vi "PTSequencer.ProcCases.vi"(0 "i ref in":refnum<vi>, 1 "selector":string, 2 "Data":T3, 3 "call cluster":T1={"Object"="", "Selector"="", "CallType"=enum."synchronous", "Async Object"="", "Async Selector"="", "Data Descriptor"="", "Data"=[], "Error #"=0, "Expire"=0}, 5 "error in (no error)":errorcluster) -> (14 "i ref out":refnum<vi>, 17 "answer cluster":T1={"Object"="", "Selector"="", "CallType"=enum."synchronous", "Async Object"="", "Async Selector"="", "Data Descriptor"="", "Data"=[], "Error #"=0, "Expire"=0}, 19 "error out":errorcluster)   [LabVIEW 2014, in "PTSequencer.lvlib"]
uses:
  PTSequencer.lvlib
  CSCore/CSSystem/CoreDefs/CoreDefs.rawDataType.ctl
  CSCore/CSSystem/CoreDefs/CoreDefs.call_type.ctl
  CSCore/BaseProcess/BaseProcess.descriptor string definition.ctl
  CSCore/CSSystem/CoreLib/CoreLib.string 2 byte array.vi
  CSCore/CSSystem/CoreLib/CoreLib.byte array 2 string.vi
  CSCore/BaseProcess/BaseProcess.lvlib
  CSCore/CAEObj/CAEObj.lvlib
  CSCore/CSSystem/CoreLib/CoreLib.lvlib
  CSCore/BaseSM/BaseSM.lvlib
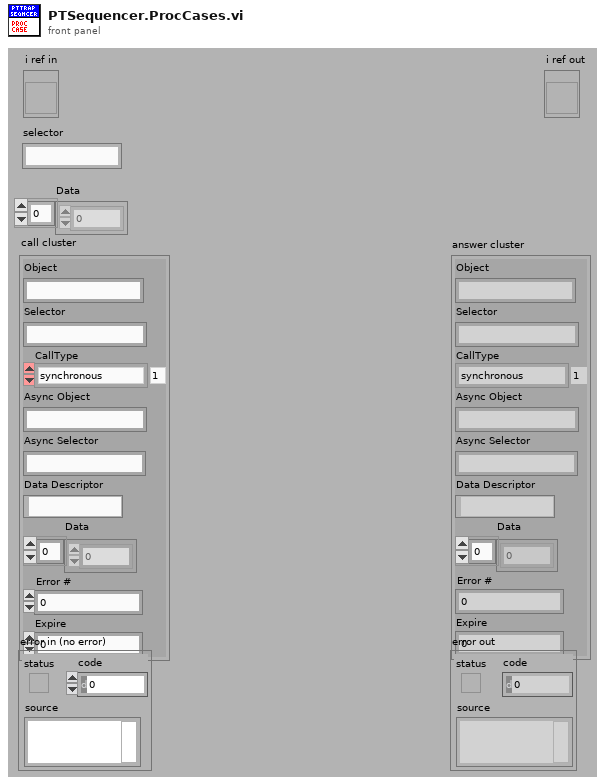
[diagram p1: front panel]
types:
  T1 = typedef "CoreDefs.call_type.ctl" = cluster{"Object":string, "Selector":string, "CallType":enum16{"simple", "synchronous", "asynchronous"}, "Async Object":string, "Async Selector":string, "Data Descriptor":T2, "Data":T3, "Error #":i32, "Expire":u32}
  T2 = typedef "BaseProcess.lvlib/BaseProcess.descriptor string definition.ctl" = string
  T3 = typedef "CoreDefs.rawDataType.ctl" = i8[]
  T4 = typedef "PTSequencer.lvlib/PTSequencer.i attribute.ctl" = cluster{"subsequence":bool, "mode":T5, "i step":i32, "nofLoops":i32, "i loop":i32, "Running":bool, "Paused":bool, "step done":bool, "loop done":bool, "seq done":bool, "DIM IDs":cluster{"step done":i32, "loop done":i32, "seq done":i32, "i step":i32, "i loop":i32}, "use stop conditions":bool, "stop conditions":T6[], "Step List":T7[], "DIM subsriptions":string[], "stop cond indexes":i32[], "step cond indexes":cluster{"step condition IDs":cluster{"step ID":i32, "condition ID":i32}[]}[], "Delay Start Time":timestamp, "status":string, "stopping":bool}
  T5 = typedef "PTSequencer.lvlib/PTSequencer.mode.ctl" = enum16{"single", "loop", "for loop"}
  T6 = typedef "PTSequencer.lvlib/PTSequencer.DIM service condition.ctl" = cluster{"DIM service":string, "descr":string, "nomValue":T3, "actValue":T3, "matched":bool, "DIM Status":cluster{"no link":bool, "quality":i32, "Time Stamp":timestamp}}
  T7 = typedef "PTSequencer.lvlib/PTSequencer.step.ctl" = cluster{"description":string, "object parameters":cluster{"object":string, "selector":string, "descriptor":string, "data":T3, "subsequence":bool, "call mode":enum16{"Simple DIM", "Synchronous"}, "data in":T3}, "result action":cluster{"check":bool, "passed":enum16{"Next", "Previous", "Repeat", "Jump"}, "failed":enum16{"Next", "Previous", "Repeat", "Jump"}, "jumpID_passed":i32, "jumpID_failed":i32}, "conditions":T6[], "fulfilled ":bool, "use delay":bool, "delay time (s)":dbl, "ID":i32}
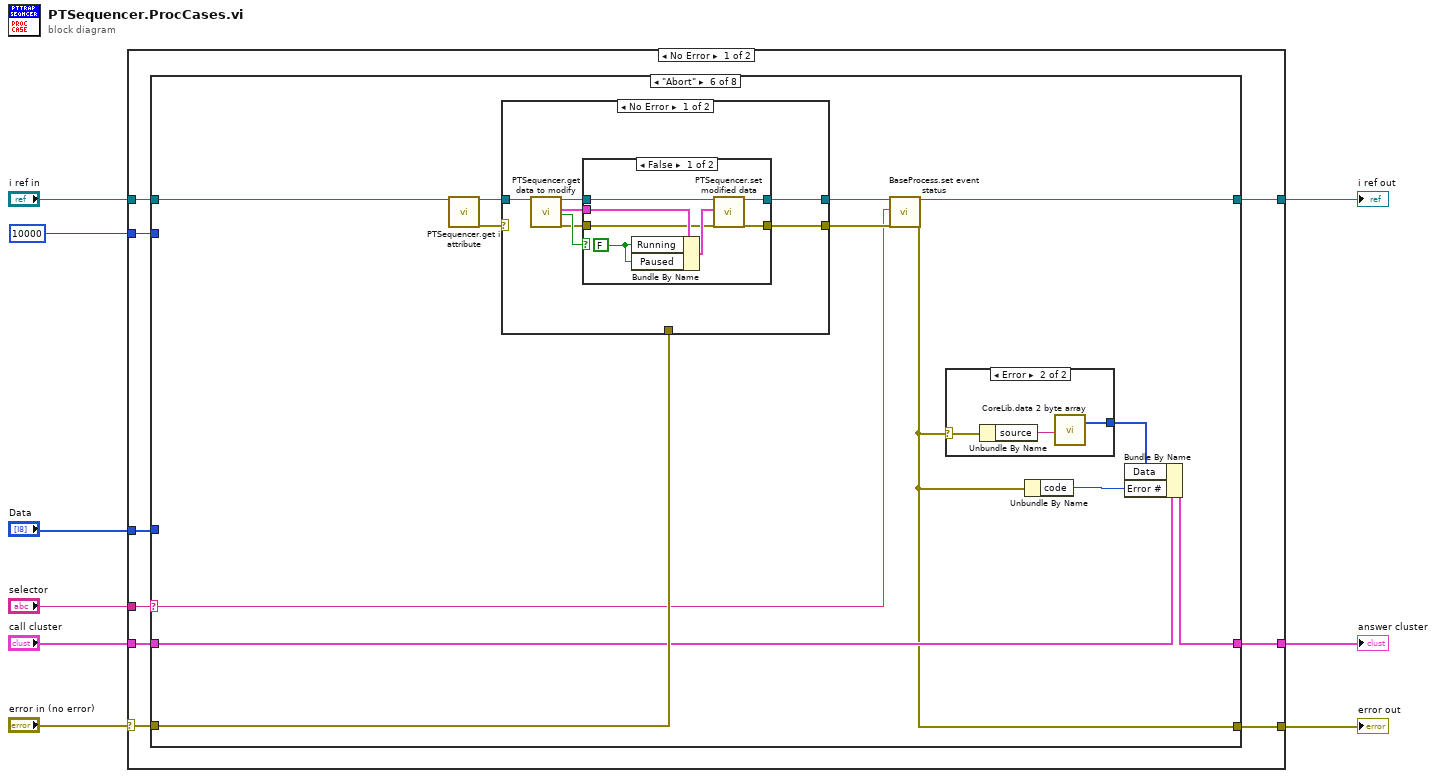
[diagram p0: block diagram]
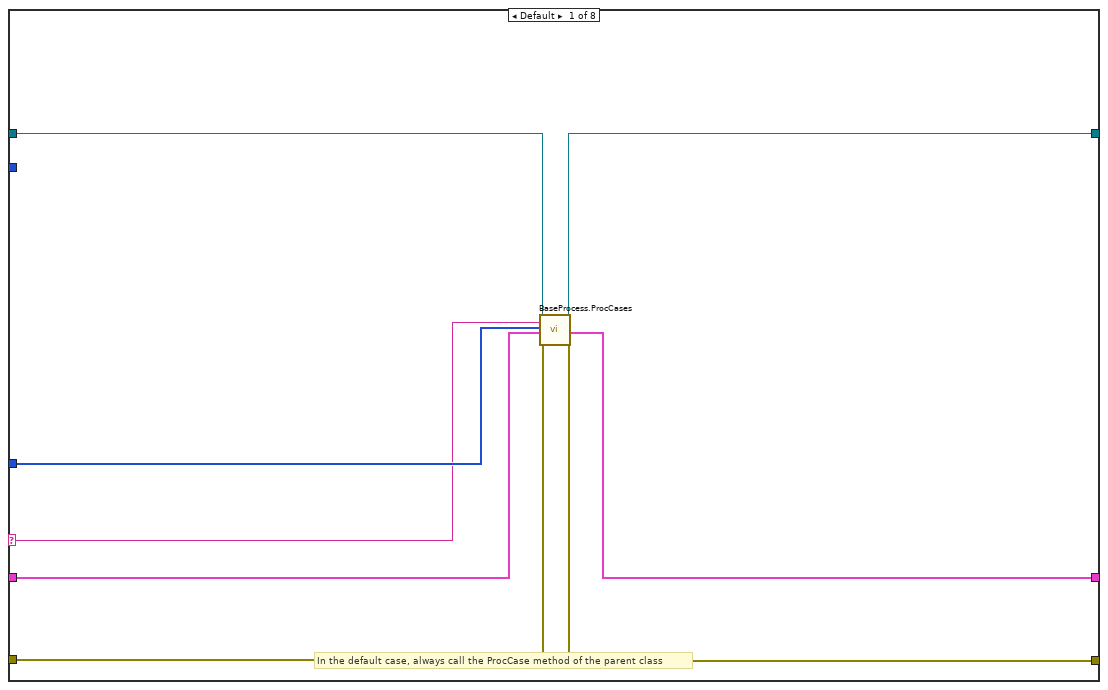
[diagram p2: hidden frame]
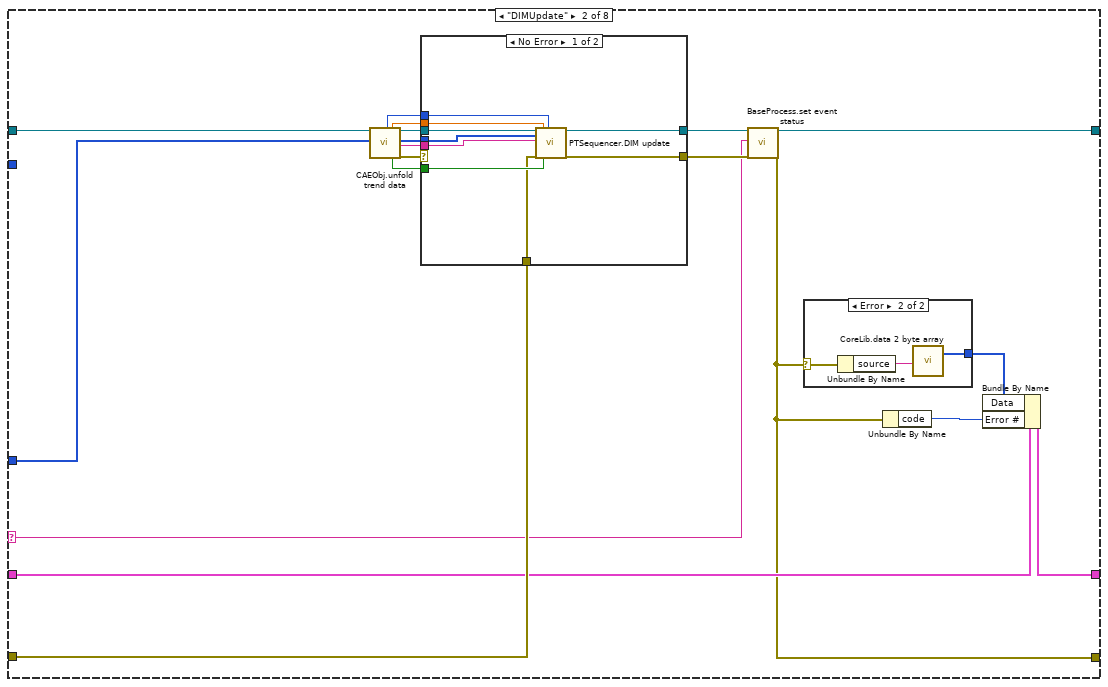
[diagram p3: hidden frame]
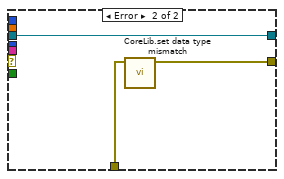
[diagram p5: hidden frame]
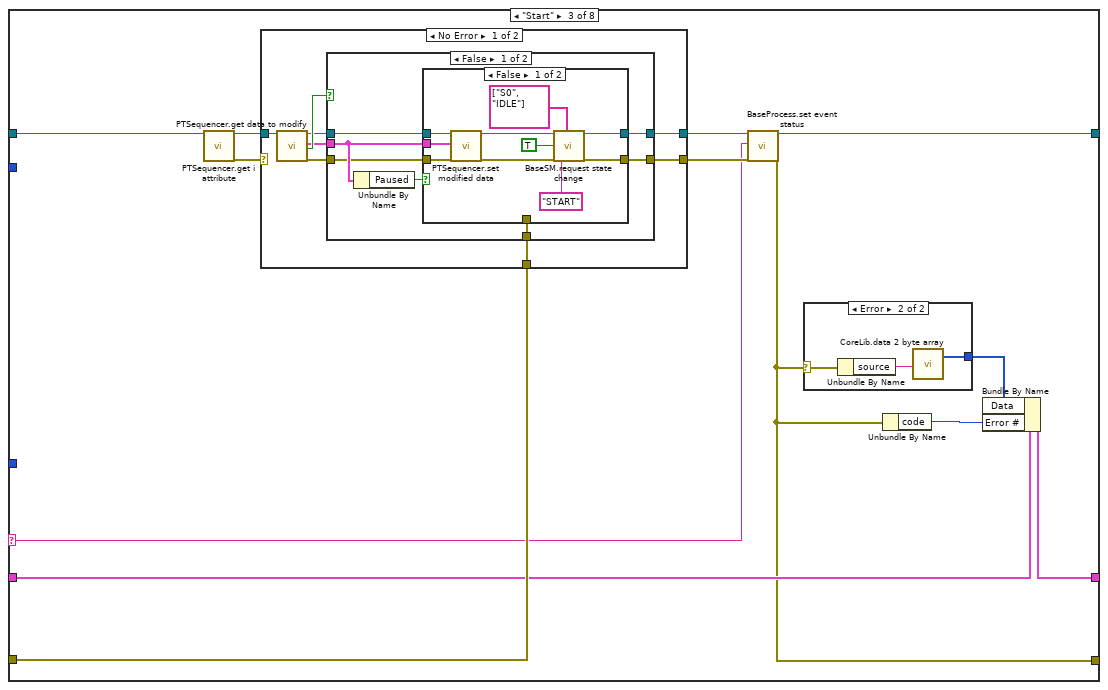
[diagram p6: hidden frame]
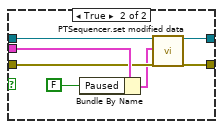
[diagram p8: hidden frame]
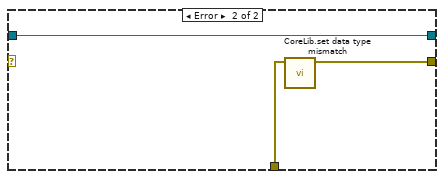
[diagram p10: hidden frame]
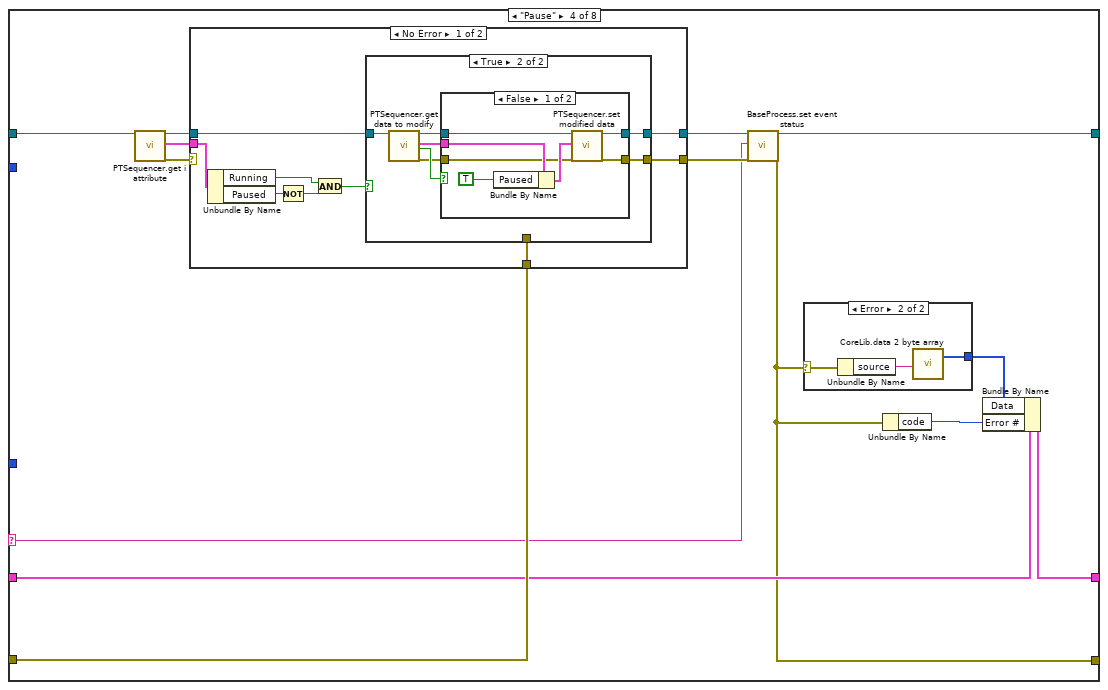
[diagram p11: hidden frame]
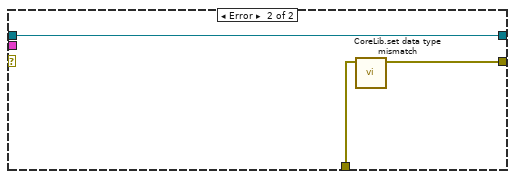
[diagram p15: hidden frame]
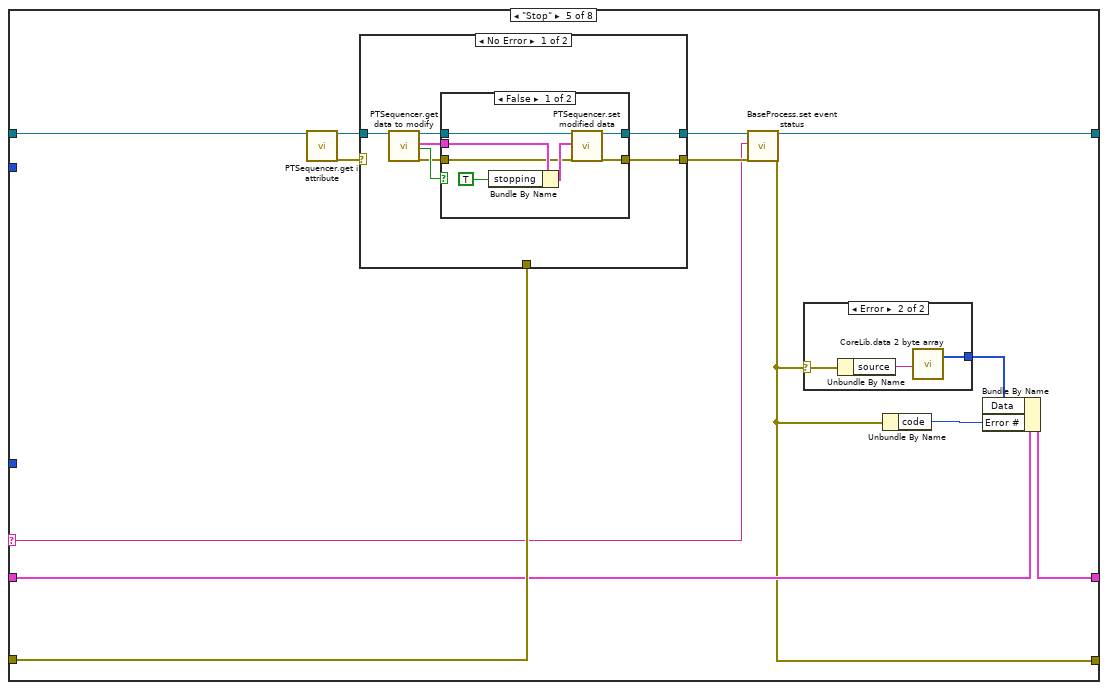
[diagram p16: hidden frame]
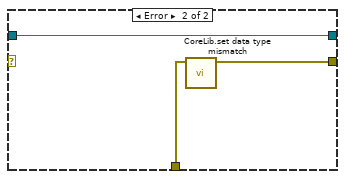
[diagram p19: hidden frame]
diagram:
  n1 = case shown="No Error" "error in (no error)" {
    selector: "error in (no error)" -> [w10 w281]
    tunnel: "selector" -> [w18 _]
    tunnel: [w17 w282] -> w8
    tunnel: "Data" -> [w16 _]
    tunnel: "call cluster" -> [w15 w282]
    tunnel: "i ref in" -> [w14 w283]
    tunnel: [w13 w283] -> w4
    tunnel: [w12 w281] -> w3
    tunnel: 10000 -> [w11 _]
    frame No Error {
      n2 = case shown="\"Abort\"" w18 {
        selector: w18 -> [w20 w30 w65 w119 w165 w200 w240 w265]
        tunnel: w16 -> [w21 w39 _ _ _ _ _ _]
        tunnel: w14 -> [w19 w29 w62 w116 w162 w197 w238 w263]
        tunnel: [w26 w28 w64 w118 w164 w199 w239 w264] -> w13
        tunnel: w15 -> [w22 w33 w68 w122 w168 w203 w234 w259]
        tunnel: [w23 w32 w67 w121 w167 w202 w242 w267] -> w17
        tunnel: w10 -> [w25 w36 w71 w125 w171 w206 w235 w260]
        tunnel: [w24 w31 w66 w120 w166 w201 w241 w266] -> w12
        tunnel: w11 -> [_ _ _ _ _ _ _ _]
        frame Default {
          # "In the default case, always call the ProcCase method of the parent class"
          n3 = call "BaseProcess.ProcCases.vi"("i ref in"=w19, "selector"=w20, "Data"=w21, "call cluster"=w22, "error in (no error)"=w25) -> ("i ref out"=w26:refnum<vi>, "answer cluster"=w23:T1, "error out"=w24:errorcluster)  [unwired: 12 in]
        }
        frame "DIMUpdate" {
          n4 = call "CAEObj.unfold trend data.vi"("i ref in"=w29, "raw trend data"=w39) -> ("quality"=w42:i32, "timeStamp"=w43:dbl, "no link"=w41:bool, "i ref out"=w27:refnum<vi>, "data"=w44:i8[], "serviceName"=w40:string, "error out"=w45:errorcluster)  [unwired: 9 in, 2 out]
          n5 = case shown="No Error" w45 {
            tunnel: w44 -> [w52 _]
            tunnel: w43 -> [w50 _]
            tunnel: w42 -> [w51 _]
            tunnel: [w55 w60] -> w34
            tunnel: w27 -> [w57 w59]
            tunnel: [w56 w59] -> w35
            tunnel: w41 -> [w54 _]
            tunnel: w40 -> [w53 _]
            tunnel: w36 -> [w49 w58]
            frame No Error {
              n6 = call "PTSequencer.DIM update.vi"("i ref in"=w57, "data"=w52, "serviceName"=w53, "error in (no error)"=w49, "Time Stamp"=w50, "no link"=w54, "quality"=w51) -> ("i ref out"=w56:refnum<vi>, "error out"=w55:errorcluster)  [unwired: 11 in]
            }
            frame Error {
              n7 = call "CoreLib.set data type mismatch.vi"("error in (no error)"=w58) -> ("error out"=w60:errorcluster)  [unwired: 18 in]
            }
          }
          n8 = call "BaseProcess.set event status.vi"("i ref in"=w35, "EventStatus"=w30, "error in (no error)"=w34) -> ("i ref out"=w28:refnum<vi>, "error out"=w31:errorcluster)  [unwired: 14 in, 1 out]
          n9 = case shown="Error" w31 {
            selector: w31 -> [_ w48]
            tunnel: [_ w46] -> w37
            frame No Error {
            }
            frame Error {
              n10 = Unbundle By Name(w48) -> ("source"=w47:string)
              n11 = call-poly "CoreLib.data 2 byte array.vi"("string"=w47) -> ("byteArray out"=w46:T3)  [unwired: 18 in]
            }
          }
          n12 = Unbundle By Name(w31) -> ("code"=w38:i32)
          n13 = Bundle By Name(cluster=w33, "Data"=w37, "Error #"=w38) -> (w32:T1)
        }
        frame "Start" {
          n14 = call "PTSequencer.get i attribute.vi"("i ref in"=w62) -> ("i ref out"=w61:refnum<vi>, "error out"=w63:errorcluster)  [unwired: 16 in, 1 out]
          n15 = case shown="No Error" w63 {
            tunnel: [w83 w113] -> w69
            tunnel: w61 -> [w81 w112]
            tunnel: [w84 w112] -> w70
            tunnel: w71 -> [w82 w111]
            frame No Error {
              n16 = call "PTSequencer.get data to modify.vi"("i ref in"=w81) -> ("i ref out"=w79:refnum<vi>, "i attribute"=w77:T4, "timed out"=w80:bool, "error out"=w78:errorcluster)  [unwired: 15 in]
              n17 = case shown="False" w80 {
                tunnel: [w91 w110] -> w84
                tunnel: [w90 w109] -> w83
                tunnel: w82 -> [w89 _]
                tunnel: w79 -> [w87 w110]
                tunnel: w78 -> [w85 w109]
                tunnel: w77 -> [w86 _]
                frame False {
                  n18 = Unbundle By Name(w86) -> ("Paused"=w88:bool)
                  n19 = case shown="False" w88 {
                    tunnel: [w98 w108] -> w91
                    tunnel: [w97 w104] -> w90
                    tunnel: w89 -> [_ _]
                    tunnel: w87 -> [w96 w107]
                    tunnel: w86 -> [w95 w106]
                    tunnel: w85 -> [w94 w105]
                    frame False {
                      n20 = call "PTSequencer.set modified data.vi"("i ref in"=w96, "CLASS.i attribute"=w95, "error in (no error)"=w94) -> ("i ref out"=w92:refnum<vi>, "error out"=w93:errorcluster)  [unwired: 15 in]
                      n21 = call "BaseSM.request state change.vi"("i ref in"=w92, "change"=TRUE, "error in (no error)"=w93, "requested state"="START", "allowed current states"=string[] ["S0", "IDLE"]) -> ("i ref out"=w98:refnum<vi>, "error out"=w97:errorcluster)  [unwired: 11 in, 2 out]
                    }
                    frame True {
                      n22 = Bundle By Name(cluster=w106, "Paused"=FALSE) -> (w103:T4)
                      n23 = call "PTSequencer.set modified data.vi"("i ref in"=w107, "CLASS.i attribute"=w103, "error in (no error)"=w105) -> ("i ref out"=w108:refnum<vi>, "error out"=w104:errorcluster)  [unwired: 15 in]
                    }
                  }
                }
                frame True {
                }
              }
            }
            frame Error {
              n24 = call "CoreLib.set data type mismatch.vi"("error in (no error)"=w111) -> ("error out"=w113:errorcluster)  [unwired: 18 in]
            }
          }
          n25 = call "BaseProcess.set event status.vi"("i ref in"=w70, "EventStatus"=w65, "error in (no error)"=w69) -> ("i ref out"=w64:refnum<vi>, "error out"=w66:errorcluster)  [unwired: 14 in, 1 out]
          n26 = case shown="Error" w66 {
            selector: w66 -> [_ w76]
            tunnel: [_ w74] -> w72
            frame No Error {
            }
            frame Error {
              n27 = Unbundle By Name(w76) -> ("source"=w75:string)
              n28 = call-poly "CoreLib.data 2 byte array.vi"("string"=w75) -> ("byteArray out"=w74:T3)  [unwired: 18 in]
            }
          }
          n29 = Unbundle By Name(w66) -> ("code"=w73:i32)
          n30 = Bundle By Name(cluster=w68, "Data"=w72, "Error #"=w73) -> (w67:T1)
        }
        frame "Pause" {
          n31 = call "PTSequencer.get i attribute.vi"("i ref in"=w116) -> ("i ref out"=w115:refnum<vi>, "i attribute"=w114:T4, "error out"=w117:errorcluster)  [unwired: 16 in]
          n32 = case shown="No Error" w117 {
            tunnel: [w138 w160] -> w123
            tunnel: w115 -> [w131 w159]
            tunnel: [w139 w159] -> w124
            tunnel: w125 -> [w137 w158]
            tunnel: w114 -> [w136 _]
            frame No Error {
              n33 = Unbundle By Name(w136) -> ("Running"=w133:bool, "Paused"=w135:bool)
              n34 = Not(x=w135) -> (.not. x?=w134:bool)
              n35 = And(x=w133, y=w134) -> (x .and. y?=w132:bool)
              n36 = case shown="True" w132 {
                tunnel: w131 -> [w141 w148]
                tunnel: [w141 w145] -> w139
                tunnel: [w140 w142] -> w138
                tunnel: w137 -> [w140 _]
                frame False {
                }
                frame True {
                  n37 = call "PTSequencer.get data to modify.vi"("i ref in"=w148) -> ("i ref out"=w146:refnum<vi>, "i attribute"=w147:T4, "timed out"=w144:bool, "error out"=w143:errorcluster)  [unwired: 15 in]
                  n38 = case shown="False" w144 {
                    tunnel: w147 -> [w155 _]
                    tunnel: w146 -> [w154 w157]
                    tunnel: [w153 w157] -> w145
                    tunnel: w143 -> [w150 w156]
                    tunnel: [w149 w156] -> w142
                    frame False {
                      n39 = Bundle By Name(cluster=w155, "Paused"=TRUE) -> (w151:T4)
                      n40 = call "PTSequencer.set modified data.vi"("i ref in"=w154, "CLASS.i attribute"=w151, "error in (no error)"=w150) -> ("i ref out"=w153:refnum<vi>, "error out"=w149:errorcluster)  [unwired: 15 in]
                    }
                    frame True {
                    }
                  }
                }
              }
            }
            frame Error {
              n41 = call "CoreLib.set data type mismatch.vi"("error in (no error)"=w158) -> ("error out"=w160:errorcluster)  [unwired: 18 in]
            }
          }
          n42 = call "BaseProcess.set event status.vi"("i ref in"=w124, "EventStatus"=w119, "error in (no error)"=w123) -> ("i ref out"=w118:refnum<vi>, "error out"=w120:errorcluster)  [unwired: 14 in, 1 out]
          n43 = case shown="Error" w120 {
            selector: w120 -> [_ w130]
            tunnel: [_ w128] -> w126
            frame No Error {
            }
            frame Error {
              n44 = Unbundle By Name(w130) -> ("source"=w129:string)
              n45 = call-poly "CoreLib.data 2 byte array.vi"("string"=w129) -> ("byteArray out"=w128:T3)  [unwired: 18 in]
            }
          }
          n46 = Unbundle By Name(w120) -> ("code"=w127:i32)
          n47 = Bundle By Name(cluster=w122, "Data"=w126, "Error #"=w127) -> (w121:T1)
        }
        frame "Stop" {
          n48 = call "PTSequencer.get i attribute.vi"("i ref in"=w162) -> ("i ref out"=w161:refnum<vi>, "error out"=w163:errorcluster)  [unwired: 16 in, 1 out]
          n49 = case shown="No Error" w163 {
            tunnel: [w177 w195] -> w169
            tunnel: w161 -> [w183 w194]
            tunnel: [w182 w194] -> w170
            tunnel: w171 -> [_ w193]
            frame No Error {
              n50 = call "PTSequencer.get data to modify.vi"("i ref in"=w183) -> ("i ref out"=w180:refnum<vi>, "i attribute"=w181:T4, "timed out"=w179:bool, "error out"=w178:errorcluster)  [unwired: 15 in]
              n51 = case shown="False" w179 {
                tunnel: w181 -> [w190 _]
                tunnel: w180 -> [w189 w192]
                tunnel: [w188 w192] -> w182
                tunnel: w178 -> [w185 w191]
                tunnel: [w184 w191] -> w177
                frame False {
                  n52 = Bundle By Name(cluster=w190, "stopping"=TRUE ("Paused")) -> (w186:T4)
                  n53 = call "PTSequencer.set modified data.vi"("i ref in"=w189, "CLASS.i attribute"=w186, "error in (no error)"=w185) -> ("i ref out"=w188:refnum<vi>, "error out"=w184:errorcluster)  [unwired: 15 in]
                }
                frame True {
                }
              }
            }
            frame Error {
              n54 = call "CoreLib.set data type mismatch.vi"("error in (no error)"=w193) -> ("error out"=w195:errorcluster)  [unwired: 18 in]
            }
          }
          n55 = call "BaseProcess.set event status.vi"("i ref in"=w170, "EventStatus"=w165, "error in (no error)"=w169) -> ("i ref out"=w164:refnum<vi>, "error out"=w166:errorcluster)  [unwired: 14 in, 1 out]
          n56 = case shown="Error" w166 {
            selector: w166 -> [_ w176]
            tunnel: [_ w174] -> w172
            frame No Error {
            }
            frame Error {
              n57 = Unbundle By Name(w176) -> ("source"=w175:string)
              n58 = call-poly "CoreLib.data 2 byte array.vi"("string"=w175) -> ("byteArray out"=w174:T3)  [unwired: 18 in]
            }
          }
          n59 = Unbundle By Name(w166) -> ("code"=w173:i32)
          n60 = Bundle By Name(cluster=w168, "Data"=w172, "Error #"=w173) -> (w167:T1)
        }
        frame "Abort" {
          n61 = call "PTSequencer.get i attribute.vi"("i ref in"=w197) -> ("i ref out"=w196:refnum<vi>, "error out"=w198:errorcluster)  [unwired: 16 in, 1 out]
          n62 = case shown="No Error" w198 {
            tunnel: [w212 w230] -> w204
            tunnel: w196 -> [w218 w229]
            tunnel: [w217 w229] -> w205
            tunnel: w206 -> [_ w228]
            frame No Error {
              n63 = call "PTSequencer.get data to modify.vi"("i ref in"=w218) -> ("i ref out"=w215:refnum<vi>, "i attribute"=w216:T4, "timed out"=w214:bool, "error out"=w213:errorcluster)  [unwired: 15 in]
              n64 = case shown="False" w214 {
                tunnel: w216 -> [w225 _]
                tunnel: w215 -> [w224 w227]
                tunnel: [w223 w227] -> w217
                tunnel: w213 -> [w221 w226]
                tunnel: [w220 w226] -> w212
                frame False {
                  w219 = FALSE ("Paused")
                  n65 = Bundle By Name(cluster=w225, "Running"=w219, "Paused"=w219) -> (w222:T4)
                  n66 = call "PTSequencer.set modified data.vi"("i ref in"=w224, "CLASS.i attribute"=w222, "error in (no error)"=w221) -> ("i ref out"=w223:refnum<vi>, "error out"=w220:errorcluster)  [unwired: 15 in]
                }
                frame True {
                }
              }
            }
            frame Error {
              n67 = call "CoreLib.set data type mismatch.vi"("error in (no error)"=w228) -> ("error out"=w230:errorcluster)  [unwired: 18 in]
            }
          }
          n68 = call "BaseProcess.set event status.vi"("i ref in"=w205, "EventStatus"=w200, "error in (no error)"=w204) -> ("i ref out"=w199:refnum<vi>, "error out"=w201:errorcluster)  [unwired: 14 in, 1 out]
          n69 = case shown="Error" w201 {
            selector: w201 -> [_ w211]
            tunnel: [_ w209] -> w207
            frame No Error {
            }
            frame Error {
              n70 = Unbundle By Name(w211) -> ("source"=w210:string)
              n71 = call-poly "CoreLib.data 2 byte array.vi"("string"=w210) -> ("byteArray out"=w209:T3)  [unwired: 18 in]
            }
          }
          n72 = Unbundle By Name(w201) -> ("code"=w208:i32)
          n73 = Bundle By Name(cluster=w203, "Data"=w207, "Error #"=w208) -> (w202:T1)
        }
        frame "SaveSettings" {
          n74 = Unbundle By Name(w234) -> ("Data"=w233:T3)
          n75 = call-poly "CoreLib.byte array 2 data.vi"("byteArray"=w233) -> ("string"=w231:string, "error out"=w232:errorcluster)  [unwired: 16 in, 1 out]
          n76 = case shown="No Error" w232 {
            tunnel: w238 -> [w249 w250]
            tunnel: [w248 w250] -> w237
            tunnel: [w247 w251] -> w236
            tunnel: w235 -> [w246 w252]
            tunnel: w231 -> [w245 _]
            frame No Error {
              n77 = call "PTSequencer.save settings.vi"("i ref in"=w249, "path"=w245, "error in (no error)"=w246) -> ("i ref out"=w248:refnum<vi>, "error out"=w247:errorcluster)  [unwired: 14 in, 1 out]
            }
            frame Error {
              n78 = call "CoreLib.set data type mismatch.vi"("error in (no error)"=w252) -> ("error out"=w251:errorcluster)  [unwired: 18 in]
            }
          }
          n79 = call "BaseProcess.set event status.vi"("i ref in"=w237, "EventStatus"=w240, "error in (no error)"=w236) -> ("i ref out"=w239:refnum<vi>, "error out"=w241:errorcluster)  [unwired: 14 in, 1 out]
          n80 = case shown="Error" w241 {
            selector: w241 -> [_ w255]
            tunnel: [_ w253] -> w243
            frame No Error {
            }
            frame Error {
              n81 = Unbundle By Name(w255) -> ("source"=w254:string)
              n82 = call-poly "CoreLib.data 2 byte array.vi"("string"=w254) -> ("byteArray out"=w253:T3)  [unwired: 18 in]
            }
          }
          n83 = Unbundle By Name(w241) -> ("code"=w244:i32)
          n84 = Bundle By Name(cluster=w234, "Data"=w243, "Error #"=w244) -> (w242:T1)
        }
        frame "LoadSettings" {
          n85 = Unbundle By Name(w259) -> ("Data"=w258:T3)
          n86 = call-poly "CoreLib.byte array 2 data.vi"("byteArray"=w258) -> ("string"=w256:string, "error out"=w257:errorcluster)  [unwired: 16 in, 1 out]
          n87 = case shown="No Error" w257 {
            tunnel: w263 -> [w274 w275]
            tunnel: [w273 w275] -> w262
            tunnel: [w272 w276] -> w261
            tunnel: w260 -> [w271 w277]
            tunnel: w256 -> [w270 _]
            frame No Error {
              n88 = call "PTSequencer.load settings.vi"("i ref in"=w274, "path"=w270, "error in (no error)"=w271) -> ("i ref out"=w273:refnum<vi>, "error out"=w272:errorcluster)  [unwired: 14 in, 1 out]
            }
            frame Error {
              n89 = call "CoreLib.set data type mismatch.vi"("error in (no error)"=w277) -> ("error out"=w276:errorcluster)  [unwired: 18 in]
            }
          }
          n90 = call "BaseProcess.set event status.vi"("i ref in"=w262, "EventStatus"=w265, "error in (no error)"=w261) -> ("i ref out"=w264:refnum<vi>, "error out"=w266:errorcluster)  [unwired: 14 in, 1 out]
          n91 = case shown="Error" w266 {
            selector: w266 -> [_ w280]
            tunnel: [_ w278] -> w268
            frame No Error {
            }
            frame Error {
              n92 = Unbundle By Name(w280) -> ("source"=w279:string)
              n93 = call-poly "CoreLib.data 2 byte array.vi"("string"=w279) -> ("byteArray out"=w278:T3)  [unwired: 18 in]
            }
          }
          n94 = Unbundle By Name(w266) -> ("code"=w269:i32)
          n95 = Bundle By Name(cluster=w259, "Data"=w268, "Error #"=w269) -> (w267:T1)
        }
      }
    }
    frame Error {
    }
  }
  "answer cluster" <- w8
  "i ref out" <- w4
  "error out" <- w3
